vi "AsciiStringToUnicodeArray.vi"(11 "String":string) -> (3 "Out array":u8[](array[numeric]))   [LabVIEW 2019]
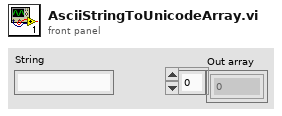
[diagram p1: front panel]
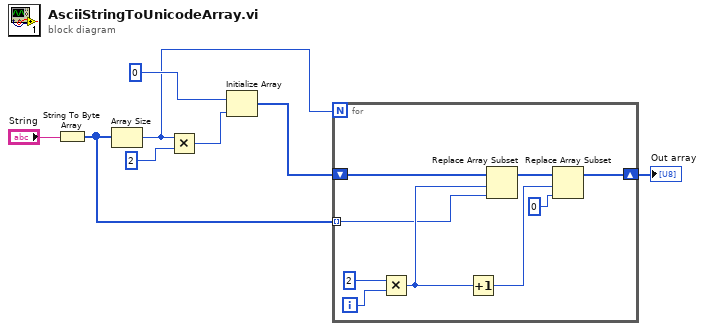
[diagram p0: block diagram]
diagram:
  n1 = String To Byte Array(string="String") -> (unsigned byte array=w2:u8[])
  n2 = Array Size(array=w2) -> (size(s)=w4:i32)
  n3 = Multiply(x=w4, y=2) -> (x*y=w6:i32)
  n4 = Initialize Array(u8 0, w6) -> (w3:u8[])
  n5 = for {
    N: w4 -> [_]
    shift-right: [w15] -> w1
    shift-left: w3 -> [w17]
    tunnel: w2 -> [w9] mode=indexing
    i -> [w14]
    n6 = Multiply(x=2, y=w14) -> (x*y=w12:i32)
    n7 = Increment(x=w12) -> (x+1=w11:i32)
    n8 = Replace Array Subset(array=w17, new element=w9, index=w12) -> (w16:u8[])
    n9 = Replace Array Subset(array=w16, new element=u8 0 ("new element/subarray"), index=w11) -> (w15:u8[])
  }
  "Out array" <- w1
